vi "Build Rx-UDP Cluster.vi"(0 "section ref in":T8=18446744073709551615 format="%.0x", 5 "board properties":T6 {"portConfig" items=["FDX_SINGLE", "FDX_REDUNDANT"]; "portSpeed" items=["FDX_100MBIT", "FDX_10MBIT", "FDX_AUTO_100MBIT", "FDX_AUTO_10MBIT", "FDX_AUTO_ERROR", "FDX_1000MBIT"]}, 9 "port properties":T5, 11 "error in":errorcluster) -> (4 "section ref out":T8 format="%.0x", 6 "boardId":u32, 8 "portId":u32, 10 "VL Configurations":T7(array[cluster]) {"VL Config"."FilterMode" items=["FDX_RX_VL_FLT_DIS", "FDX_RX_VL_FLT_ENA ", "FDX_RX_VL_FLT_ENA_INV"]; "VL Config"."VLBufSize" format="%.0x"; "VL Config"."VerificationMode" items=["FDX_RX_VL_CHECK_ENA_DEFAULT"=65535, "FDX_RX_VL_CHECK_REDMAM"=16, "DX_RX_VL_CHECK_TRAFIC"=8, "FDX_RX_VL_CHECK_FRAMESIZE"=4, "FDX_RX_VL_CHECK_SNINTEG"=2, "FDX_RX_VL_CHECK_INVPAC"=1, "FDX_RX_VL_CHECK_DISA"=0]}, 14 "CommPort Payload":T4(array[cluster]), 15 "error out":errorcluster)   [LabVIEW 2020, in "AIM ARINC 664 Scripting.lvlib"]
uses:
  AIM ARINC 664 Scripting.lvlib
  <vilib>/NI VeriStand/Custom Device API/Custom Device Item Ref.ctl
  <instrlib>/AIM GmbH/_AIM 664/_controls/comm_verification_rx.ctl
  <instrlib>/AIM GmbH/_AIM 664/_controls/comm_udp_rx.ctl
  Shared/board_setup.ctl
  Shared/port_setup.ctl
  <vilib>/NI/NI VeriStand Encoding and Decoding/Encoding.ctl
  <vilib>/NI VeriStand/Custom Device API/Custom Device API.lvlib
  <instrlib>/AIM GmbH/_AIM 664/AIM664LV.lvlib
  <vilib>/NI/NI VeriStand Encoding and Decoding/Encoding and Decoding.lvlib
  <vilib>/Utility/SystemLogging/NI_SystemLogging.lvlib
  Import/AIM ARINC 664 Import.lvlib
panel:
  in  "Cluster":cluster{"VL Config":T1, "CommPort Config":T2[]} {"VL Config"."FilterMode" items=["FDX_RX_VL_FLT_DIS", "FDX_RX_VL_FLT_ENA ", "FDX_RX_VL_FLT_ENA_INV"]; "VL Config"."VLBufSize" format="%.0x"; "VL Config"."VerificationMode" items=["FDX_RX_VL_CHECK_ENA_DEFAULT"=65535, "FDX_RX_VL_CHECK_REDMAM"=16, "DX_RX_VL_CHECK_TRAFIC"=8, "FDX_RX_VL_CHECK_FRAMESIZE"=4, "FDX_RX_VL_CHECK_SNINTEG"=2, "FDX_RX_VL_CHECK_INVPAC"=1, "FDX_RX_VL_CHECK_DISA"=0]}
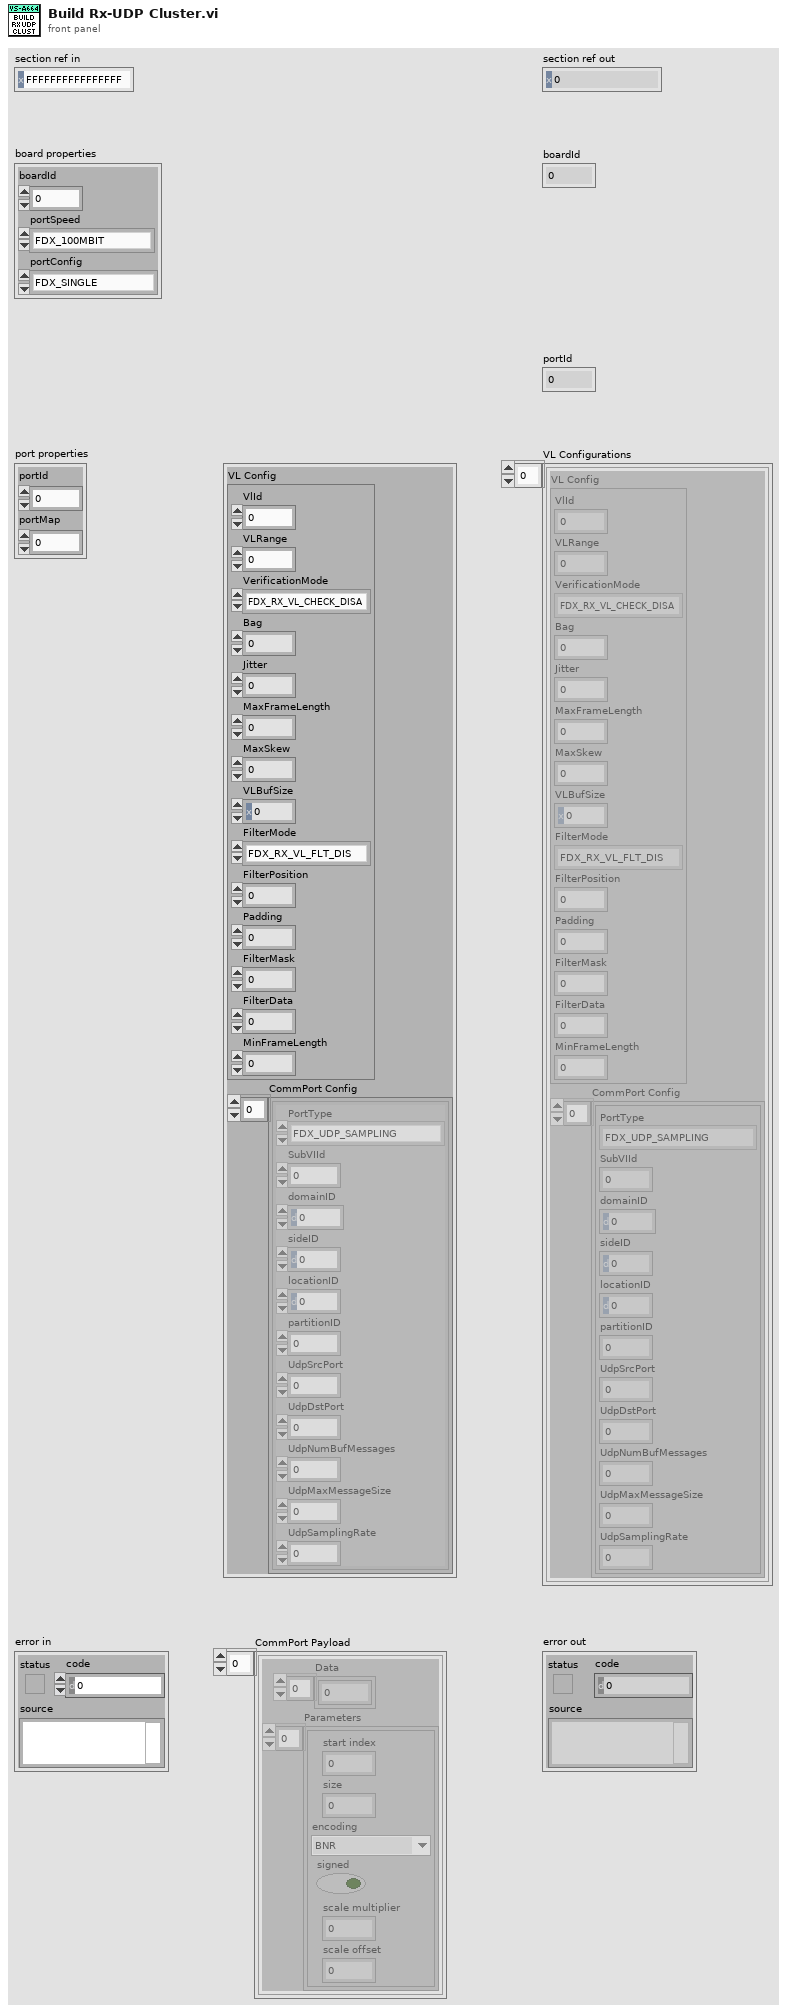
[diagram p1: front panel]
types:
  T1 = typedef "AIM664LV.lvlib/comm_verification_rx.ctl" = cluster{"VlId":u16, "VLRange":u32, "VerificationMode":u32, "Bag":u32, "Jitter":u32, "MaxFrameLength":u32, "MaxSkew":u32, "VLBufSize":u32, "FilterMode":u32, "FilterPosition":u32, "Padding":u32, "FilterMask":u32, "FilterData":u32, "MinFrameLength":u32}
  T2 = typedef "AIM664LV.lvlib/comm_udp_rx.ctl" = cluster{"PortType":enum16{"FDX_UDP_SAMPLING", "FDX_UDP_QUEUING"}, "SubVIId":u32, "domainID":u8, "sideID":u8, "locationID":u8, "partitionID":u8, "UdpSrcPort":u16, "UdpDstPort":u16, "UdpNumBufMessages":u32, "UdpMaxMessageSize":u32, "UdpSamplingRate":u32}
  T3 = typedef "Encoding and Decoding.lvlib/Encoding.ctl" = enum16{"BNR", "BCD", "Discrete"}
  T4 = cluster{"Data":u8[], "Parameters":cluster{"start index":i32, "size":i32, "encoding":T3, "signed":bool, "scale multiplier":dbl, "scale offset":dbl}[]}[]
  T5 = typedef "AIM ARINC 664 Import.lvlib/port_setup.ctl" = cluster{"portId":u32, "portMap":u32}
  T6 = typedef "AIM ARINC 664 Import.lvlib/board_setup.ctl" = cluster{"boardId":u32, "portSpeed":u32, "portConfig":u32}
  T7 = cluster{"VL Config":T1, "CommPort Config":T2[]}[]
  T8 = typedef "Custom Device API.lvlib/Custom Device Item Ref.ctl" = u64
  T9 = cluster{"Data":u8[], "Parameters":cluster{"start index":i32, "size":i32, "encoding":T3, "signed":bool, "scale multiplier":dbl, "scale offset":dbl}[]}
  T10 = cluster{"start index":i32, "size":i32, "encoding":T3, "signed":bool, "scale multiplier":dbl, "scale offset":dbl}
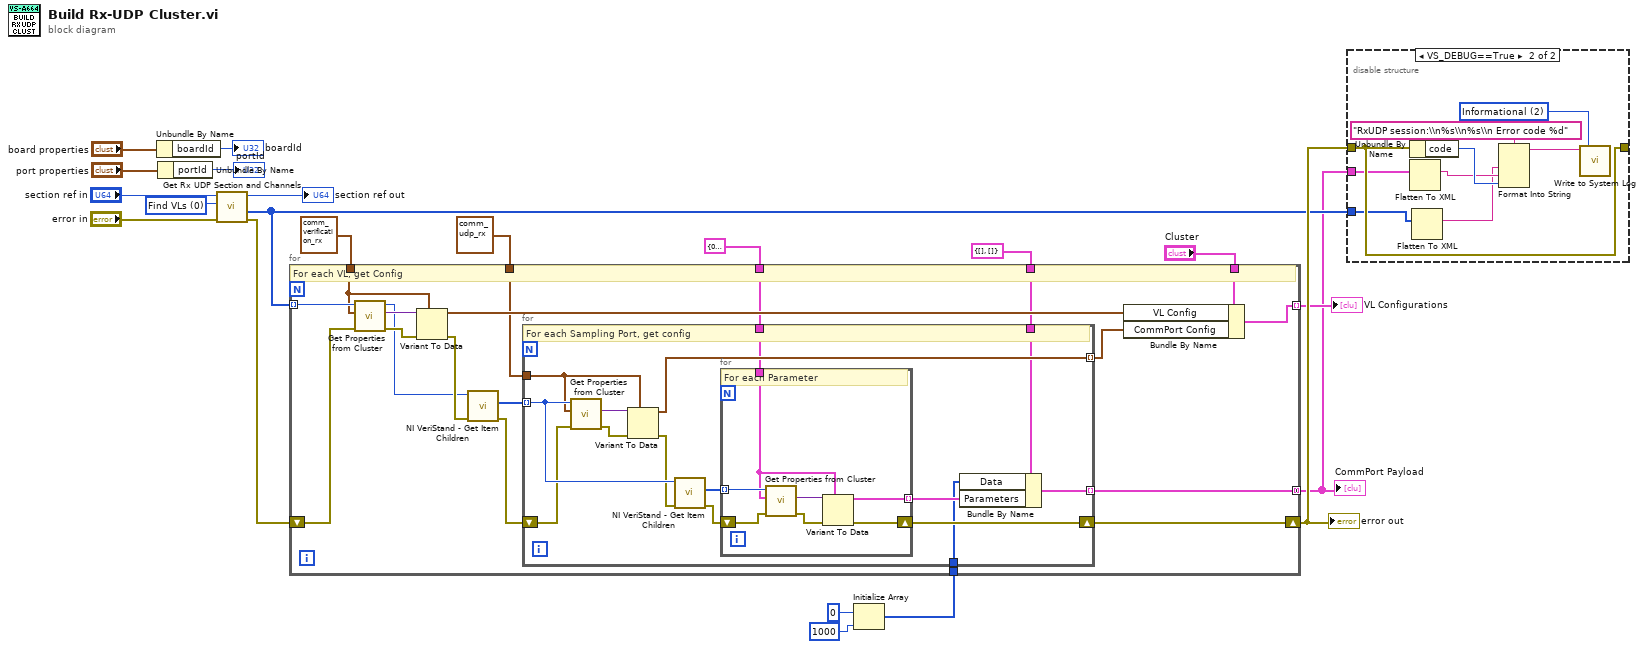
[diagram p0: block diagram]
diagram:
  w3 = u16 0 items=["Find VLs", "Find Parameters"] ("Option")
  n1 = Unbundle By Name("board properties") -> ("boardId"=→"boardId":u32)
  n2 = Unbundle By Name("port properties") -> ("portId"=→"portId":u32)
  n3 = call "Get Rx UDP Section and Channels.vi"("error in"="error in", "Option"=w3, "Custom Device Ref in"="section ref in") -> ("error out"=w6:errorcluster, "Tx Queue Status channel Refs"=w2:T8[], "Custom Device Ref out"=→"section ref out":T8)  [unwired: 4 in, 2 out]
  n4 = Initialize Array(0 ("Numeric"), 1000 ("dimension size")) -> (w12:i32[])
  n5 = for {
    tunnel: [w32] -> w8 mode=indexing
    shift-right: [w30] -> w9
    shift-left: w6 -> [w40]
    tunnel: [w23] -> w1 mode=concatenating
    tunnel: w2 -> [w29] mode=indexing
    tunnel: "Cluster" -> [w28]
    tunnel: T2 {"PortType"=enum."FDX_UDP_SAMPLING", "SubVIId"=0, "domainID"=1, "sideID"=1, "locationID"=1, "partitionID"=1, "UdpSrcPort"=0, "UdpDstPort"=0, "UdpNumBufMessages"=0, "UdpMaxMessageSize"=0, "UdpSamplingRate"=0} ("CommPort Config") -> [w27]
    tunnel: T1 {"VlId"=0, "VLRange"=0, "VerificationMode"=0, "Bag"=0, "Jitter"=0, "MaxFrameLength"=0, "MaxSkew"=0, "VLBufSize"=32768, "FilterMode"=0, "FilterPosition"=0, "Padding"=0, "FilterMask"=0, "FilterData"=0, "MinFrameLength"=0} ("VL Config") -> [w26]
    tunnel: T10 {"start index"=0, "size"=0, "encoding"=enum."BNR", "signed"=FALSE, "scale multiplier"=0.0, "scale offset"=0.0} ("Parameter") -> [w25]
    tunnel: T9 {"Data"=[], "Parameters"=[]} ("Data and Parameters") -> [w24]
    tunnel: w12 -> [w22]
    # "For each VL, get Config"
    n6 = call "Get Properties from Cluster.vi"("error in"=w40, "Variant Cluster"=w26, "custom device ref in"=w29) -> ("error out"=w38:errorcluster, "data"=w39:variant, "custom device ref out"=w36:T8)  [unwired: 5 in, 1 out]
    n7 = Variant To Data(error in=w38, type=w26, Variant=w39) -> (data=w33:T1, error out=w37:errorcluster)
    n8 = call <vilib>:"NI VeriStand - Get Item Children.vi"("error in (no error)"=w37, "Item Ref in"=w36) -> ("error out"=w34:errorcluster, "Child Refs"=w35:T8[])  [unwired: 6 in, 2 out]
    n9 = for {
      tunnel: w35 -> [w51] mode=indexing
      shift-right: [w47] -> w30
      shift-left: w34 -> [w46]
      tunnel: [w50] -> w31 mode=indexing
      tunnel: [w48] -> w23 mode=indexing
      tunnel: w27 -> [w44]
      tunnel: w25 -> [w43]
      tunnel: w24 -> [w42]
      tunnel: w22 -> [w41]
      # "For each Sampling Port, get config"
      n10 = call "Get Properties from Cluster.vi"("error in"=w46, "Variant Cluster"=w44, "custom device ref in"=w51) -> ("error out"=w53:errorcluster, "data"=w52:variant)  [unwired: 5 in, 2 out]
      n11 = Variant To Data(error in=w53, type=w44, Variant=w52) -> (data=w50:T2, error out=w45:errorcluster)
      n12 = call <vilib>:"NI VeriStand - Get Item Children.vi"("error in (no error)"=w45, "Item Ref in"=w51) -> ("error out"=w54:errorcluster, "Child Refs"=w55:T8[])  [unwired: 6 in, 2 out]
      n13 = for {
        tunnel: w55 -> [w60] mode=indexing
        shift-right: [w57] -> w47
        shift-left: w54 -> [w58]
        tunnel: [w59] -> w49 mode=indexing
        tunnel: w43 -> [w56]
        # "For each Parameter"
        n14 = call "Get Properties from Cluster.vi"("error in"=w58, "Variant Cluster"=w56, "custom device ref in"=w60) -> ("error out"=w61:errorcluster, "data"=w62:variant)  [unwired: 5 in, 2 out]
        n15 = Variant To Data(error in=w61, type=w56, Variant=w62) -> (data=w59:T10, error out=w57:errorcluster)
      }
      n16 = Bundle By Name(cluster=w42, "Data"=w41, "Parameters"=w49) -> (w48:T9)
    }
    n17 = Bundle By Name(cluster=w28, "VL Config"=w33, "CommPort Config"=w31) -> (w32:cluster{"VL Config":T1, "CommPort Config":T2[]})
  }
  "error out" <- w9
  "VL Configurations" <- w8
  "CommPort Payload" <- w1
  n18 = disable-structure shown="VS_DEBUG==True" {
    disable-tunnel: w9 -> [_ w67]
    disable-tunnel: [_ w67] -> _
    disable-tunnel: w1 -> [_ w66]
    disable-tunnel: w2 -> [_ w64]
    frame condition #0 {
    }
    frame condition #1 (active) {
      w69 = 2 items=["Error", "Warning", "Informational"] ("severity")
      n19 = Unbundle By Name(w67) -> ("code"=w68:i32)
      n20 = Flatten To XML(6:w66) -> (2:w65:string)
      n21 = Flatten To XML(6:w64) -> (2:w63:string)
      n22 = Format Into String(format string="RxUDP session:\\n%s\\n%s\\n Error code %d", w63, w65, w68) -> (resulting string=w70:string)  [unwired: 2 in, 1 out]
      n23 = call <vilib>:"Write to System Log.vi"("severity"=w69, "message"=w70) -> ()  [unwired: 9 in, 1 out]
    }
  }
